vi "Request Data JSON.vi"(8 "error in (no error)":errorcluster, 11 "SetInputVolume in":refnum<class "SetInputVolume.lvclass">) -> (0 "error out":errorcluster, 2 "Request Data JSON":string, 3 "SetInputVolume out":refnum<class "SetInputVolume.lvclass">)   [LabVIEW 2022 SP3, in "obs-websocket-lv.lvlib" / "SetInputVolume.lvclass"]
uses:
  SetInputVolume.lvclass
  SetInputVolume.lvclass/SetInputVolume.ctl
  <vilib>/IlluminatedG/lv-web-crypto/lv-json/JSON/JSON.lvlib
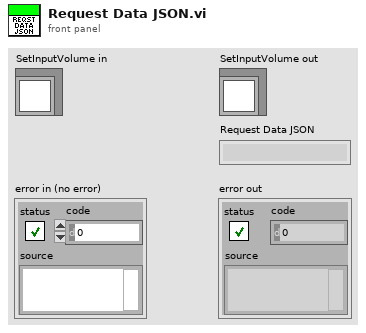
[diagram p1: front panel]
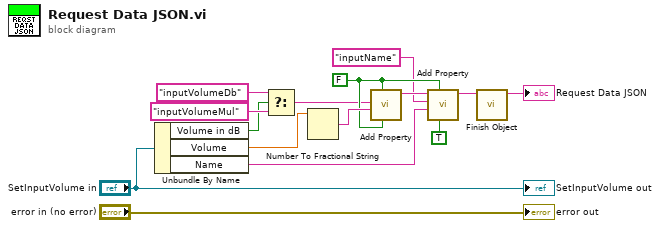
[diagram p0: block diagram]
diagram:
  w9 = FALSE ("Include Empty?")
  n1 = Unbundle By Name("SetInputVolume in") -> ("Volume in dB"=w4:bool, "Volume"=w2:dbl, "Name"=w1:string)
  n2 = Select(t="inputVolumeDb", s=w4, f="inputVolumeMul") -> (s? t:f=w3:string)
  n3 = Number To Fractional String(number=w2) -> (F-format string=w13:string)  [unwired: 3 in]
  n4 = call <vilib>:"Add Property.vi"("String?"=w9, "Include Empty?"=w9, "Value"=w13, "Property Name"=w3) -> ("String out"=w11:string)  [unwired: 7 in]
  n5 = call <vilib>:"Add Property.vi"("String?"=TRUE, "Include Empty?"=w9, "Value"=w1, "Property Name"="inputName", "String In"=w11) -> ("String out"=w10:string)  [unwired: 6 in]
  n6 = call <vilib>:"Finish Object.vi"("String In"=w10) -> ("String out"=→"Request Data JSON":string)  [unwired: 10 in]
  "error out" <- "error in (no error)"
  "SetInputVolume out" <- "SetInputVolume in"
